vi "TCP Message Interpreter.vi"(8 "error in (no error)":errorcluster, 9 "Data":variant, 10 "Message":string, 11 "Guardian in":refnum<class "Guardian.lvclass">) -> (0 "error out":errorcluster, 3 "Guardian out":refnum<class "Guardian.lvclass">)   [LabVIEW 2026, in "TALOS.lvlib" / "Guardian.lvlib" / "Guardian.lvclass"]
doc: "Use this VI to send a message to the Guardian, from the outside (i.e. from a uService). For internal messages, use the Actor Framework messages system."
uses:
  Guardian.lvclass
  C:/LabVIEW Code/TALOS/builds/Actor Framework PPL/Actor Framework.lvlibp/1abvi3w/vi.lib/ActorFramework/Actor/Actor.lvclass
  C:/LabVIEW Code/TALOS/talos/Ancestor/Ancestor/Ancestor.lvclass
  Ancestor/Ancestor/Ancestor.lvclass/Ancestor.ctl
  Guardian Messages/Ready to launch Msg/Ready to launch Msg.lvclass/Ready to launch Msg.ctl
  Father of all uServices/Father of all uServices/Event Handler Items.ctl
  Guardian.lvclass/Guardian.ctl
  Guardian Messages/Message to uService Msg/Message to uService Msg.lvclass/Message to uService Msg.ctl
  Ancestor/Ancestor/Infinite Message Selector.ctl
  Guardian Messages/Message to Other Guardian Msg/Message to Other Guardian Msg.lvclass/Message to Other Guardian Msg.ctl
  Classes/uService List/uService List.lvclass/uService List.ctl
  Git Update Cluster.ctl
  builds/Actor Framework PPL/Actor Framework.lvlibp/1abvi3w/vi.lib/ActorFramework/Message Enqueuer/Message Priority.ctl
  Guardian Messages/Raise or Lower Abort Msg/Raise or Lower Abort Msg.lvclass/Raise or Lower Abort Msg.ctl
  Ancestor/Ancestor/Read Distr uS Map ref.vi
  Ancestor/Ancestor/Write Distr uS Map ref.vi
  Ancestor/Ancestor/Read ID.vi
  Read Guardian List.vi
  Write Guardian List.vi
  FGV/Error Memory/Get Error Description.vi
  Support VIs/Get PC name.vi
  Support VIs/Get Class Name.vi
  <vilib>/Utility/error.llb/Clear Errors.vi
  Support VIs/Circus Root Path.vi
  FGV/Error Memory/Error Memory Core.vi
  <vilib>/AdvancedString/Delimited String to 1D String Array.vi
  <vilib>/AdvancedString/Delimited String to 1D String Array (string).vi
  FGV/Error Memory/Error Crt Lvl checker.vi
  FGV/Error Memory/Error Memory Core.vi/40c8088d-b597-4017-91af-faa98e00292e.vi
  FGV/Error Memory/Error Memory Core.vi/d4a3ab98-063c-4e44-b43d-fbdcfe6c2be2.vi
  Support VIs/Global Memory.vi
  <vilib>/Utility/LVClass/Get LV Class Name.vi
  Support VIs/TALOS Root path.vi
  Support VIs/Read CSV worksheet.vi
  Support VIs/Global Constants.vi
  <vilib>/Utility/error.llb/General Error Handler.vi
  builds/Actor Framework PPL/Actor Framework.lvlibp/1abvi3w/vi.lib/ActorFramework/Message Enqueuer/Enqueue.vi
  Support VIs/Error Log.vi
  <vilib>/Utility/config.llb/Open Config Data.vi
  <vilib>/Utility/config.llb/Get Section Names.vi
  <vilib>/Utility/config.llb/Get Key Names.vi
  <vilib>/Utility/config.llb/Read Key.vi
  <vilib>/Utility/config.llb/Read Key (String).vi
  <vilib>/Utility/config.llb/Close Config Data.vi
  Ancestor/Ancestor/Ancestor.lvclass
  <vilib>/Comparison/Equal/Equal Functor/Equal Functor.lvclass
  Guardian Messages/Ready to launch Msg/Ready to launch Msg.lvclass
  Guardian Messages/Message to uService Msg/Message to uService Msg.lvclass
  Guardian Messages/Message to Other Guardian Msg/Message to Other Guardian Msg.lvclass
  Classes/Distributed uService Map/Distributed uService Map.lvclass
  Classes/Guardian List/Guardian List.lvclass
  Guardian Messages/Raise or Lower Abort Msg/Raise or Lower Abort Msg.lvclass
  builds/Actor Framework PPL/Actor Framework.lvlibp/1abvi3w/vi.lib/ActorFramework/Message Enqueuer/Message Enqueuer.lvclass
  TALOS.lvlib
  Father of all uServices/Father of all uServices/Father of all uServices.lvclass
  builds/Actor Framework PPL/Actor Framework.lvlibp/1abvi3w/vi.lib/ActorFramework/Actor/Actor.lvclass
  Im alive message.ctl
  Classes/uService List/uService List.lvclass
  Classes/Error Filter/Error Filter.lvclass
  FGV/Error Memory/Error Memory.lvlib
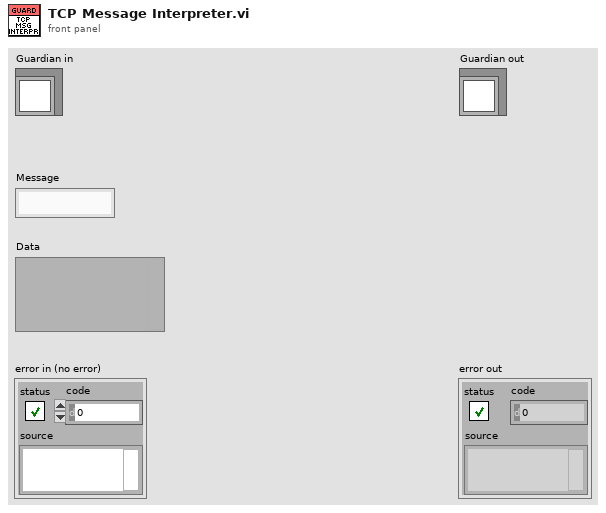
[diagram p1: front panel]
types:
  T1 = typedef "TALOS.lvlib/Father of all uServices.lvlib/Father of all uServices.lvclass/Event Handler Items.ctl" = enum16{"Button Pressed", "Message", "Ready to launch?", "Safe Mode", "Start RUN", "Stop RUN"}
  T2 = typedef "TALOS.lvlib/Ancestor.lvlib/Ancestor.lvclass/Infinite Message Selector.ctl" = enum16{"Start", "Stop", "Check", "Flush (Stop all)", "Init"}
  T3 = typedef "TALOS.lvlib/Guardian.lvlib/Guardian.lvclass/Im alive message.ctl" = cluster{"ID":string, "Time":timestamp, "Abort":bool, "Bearer":bool}
  T4 = typedef "Actor Framework.lvlibp/Message Enqueuer.lvclass/Message Priority.ctl" = enum16{"Low", "Normal", "High"}
  T5 = typedef "TALOS.lvlib/Guardian.lvlib/Guardian.lvclass/Git Update Cluster.ctl" = cluster{"branch name":string, "include critical PCs":bool, "update from git":bool}
  T6 = typedef "TALOS.lvlib/Guardian.lvlib/Guardian.lvclass/Run Config Data.ctl" = cluster{"Name":string, "uS List":string[]}
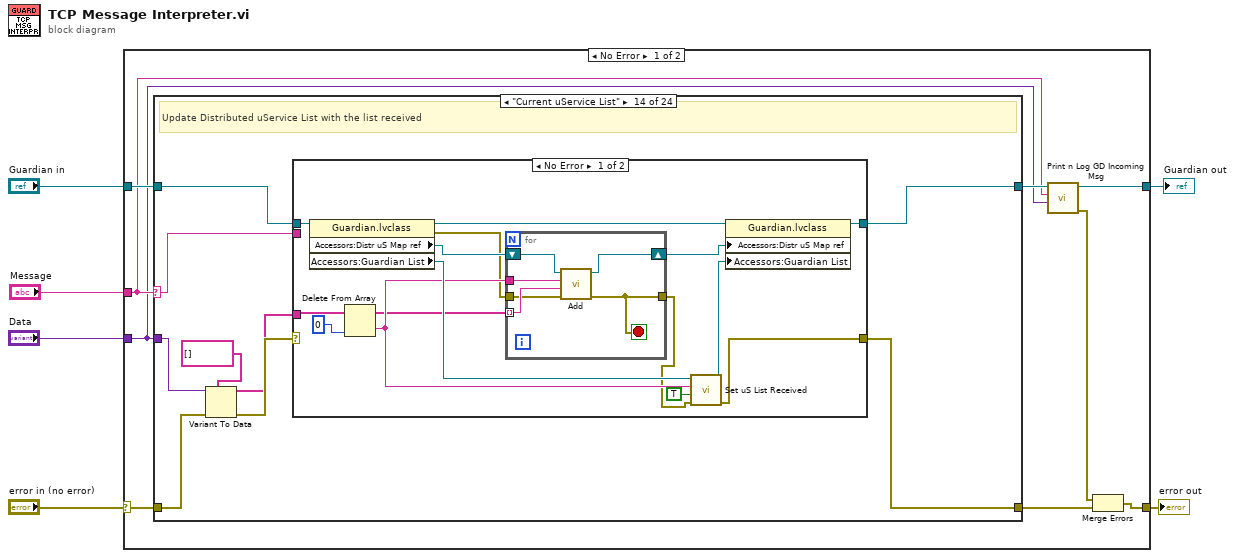
[diagram p0: block diagram]
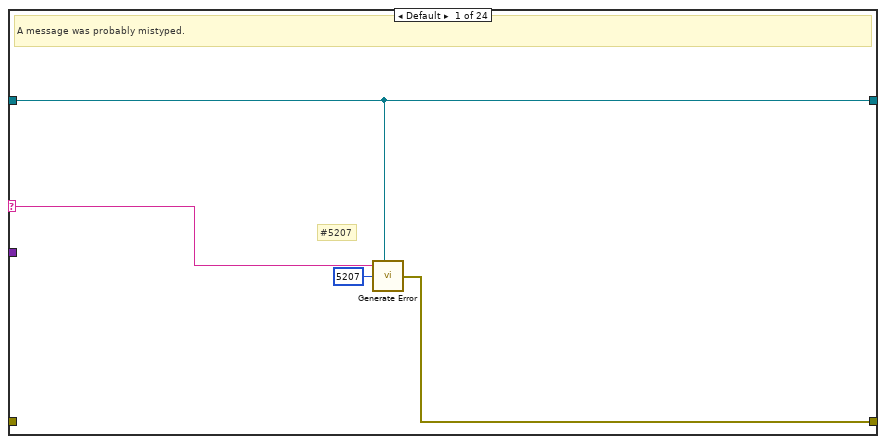
[diagram p2: hidden frame]
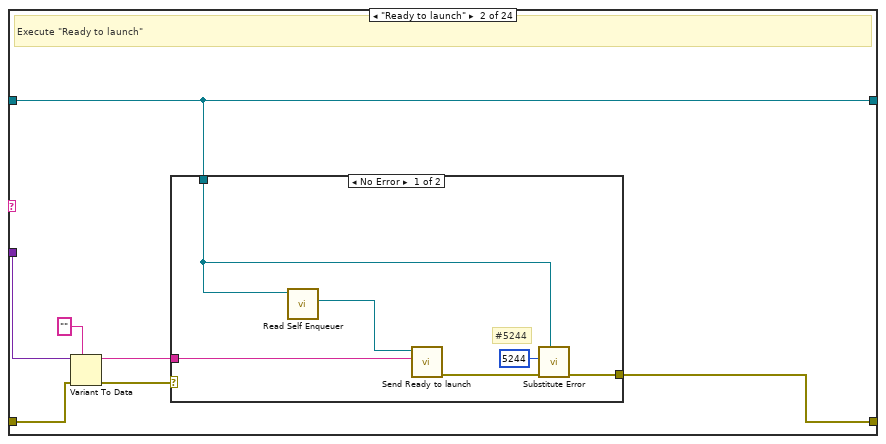
[diagram p3: hidden frame]
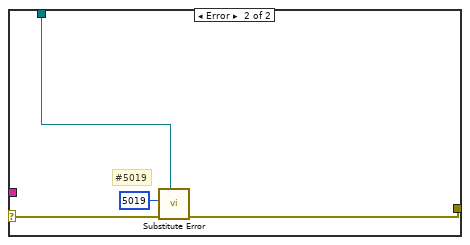
[diagram p4: hidden frame]
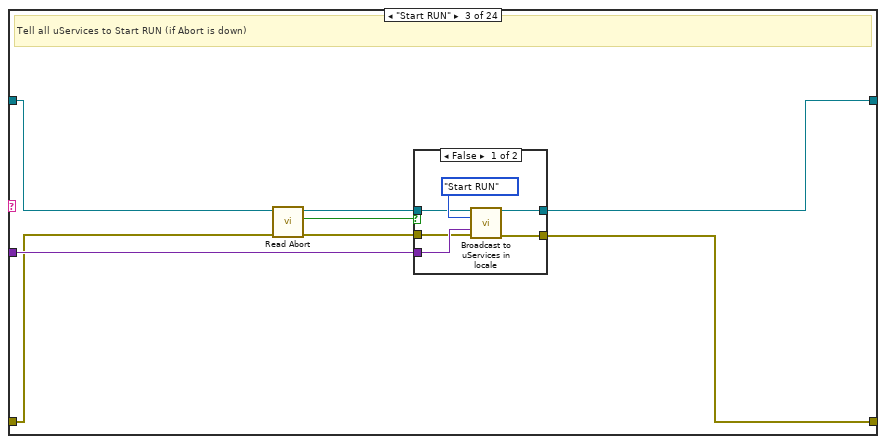
[diagram p5: hidden frame]
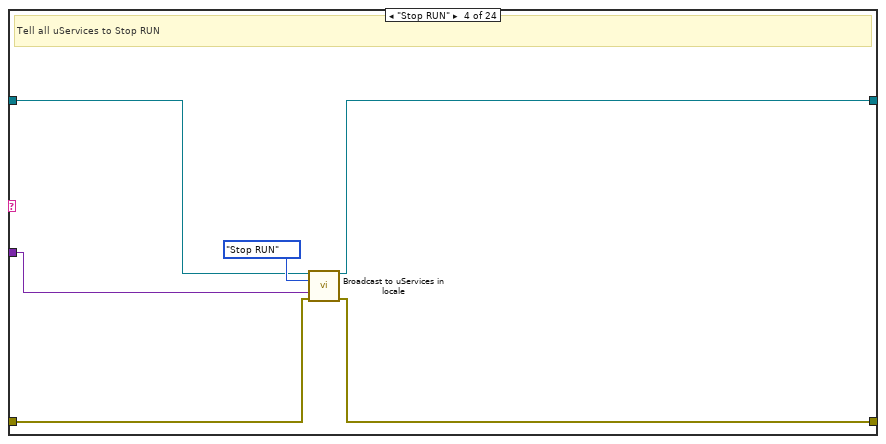
[diagram p7: hidden frame]
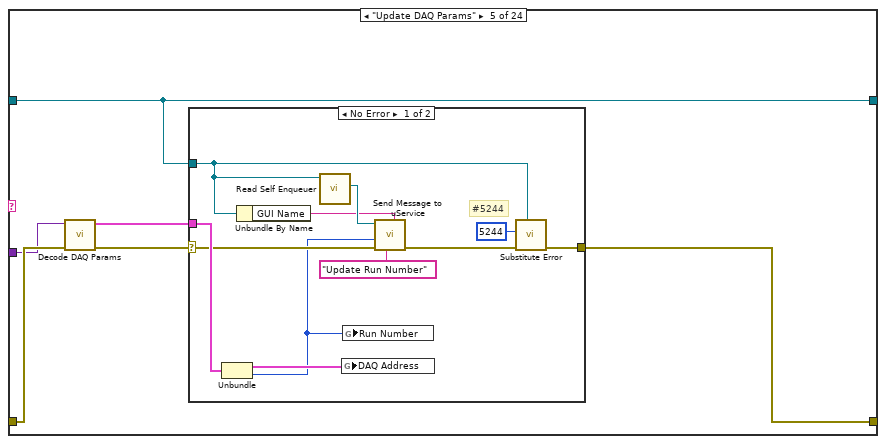
[diagram p8: hidden frame]
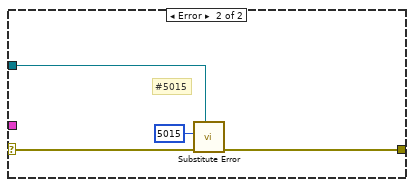
[diagram p9: hidden frame]
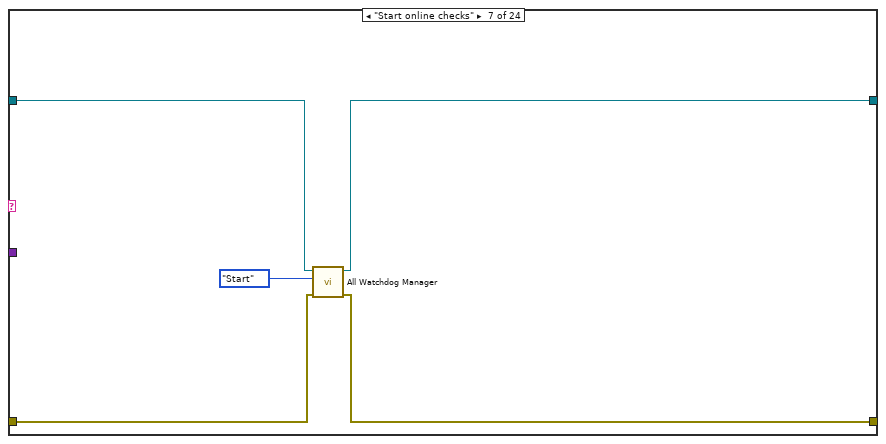
[diagram p11: hidden frame]
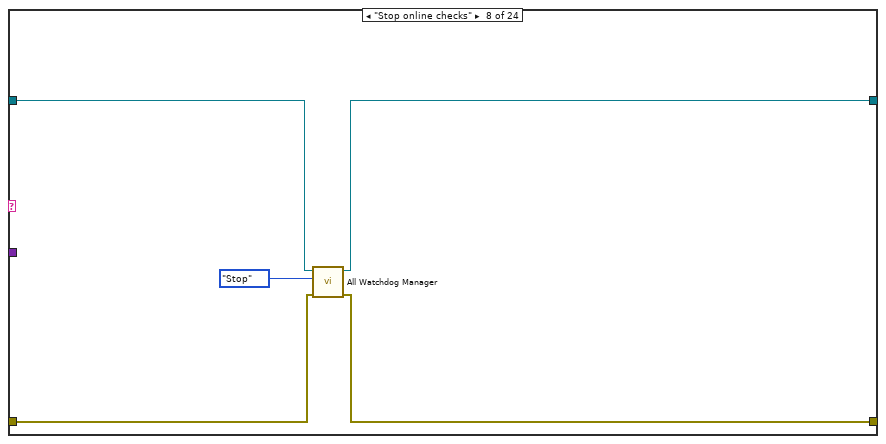
[diagram p12: hidden frame]
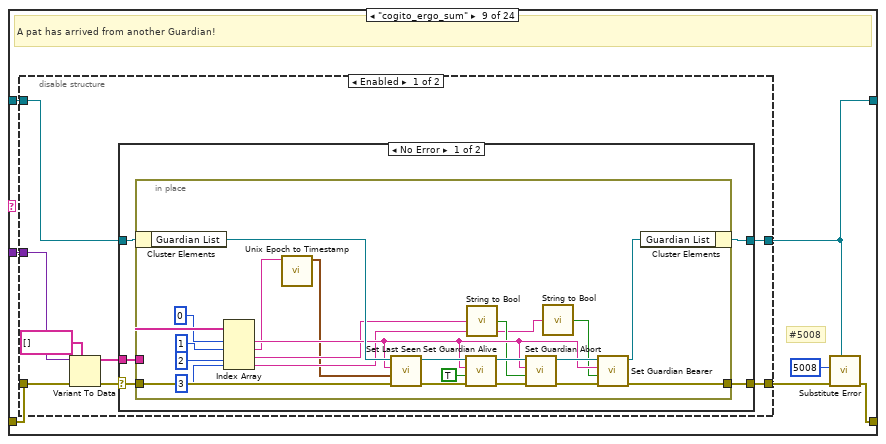
[diagram p13: hidden frame]
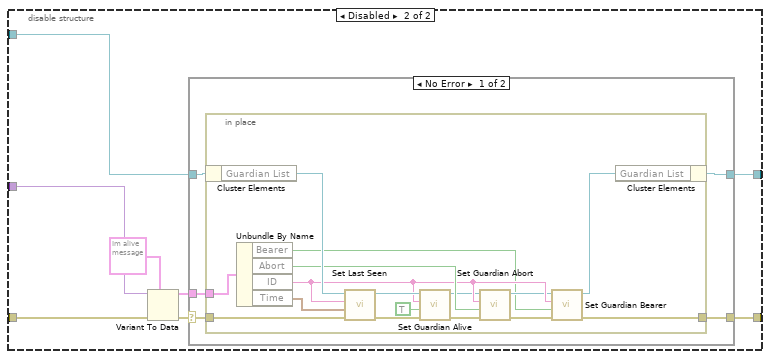
[diagram p15: hidden frame]
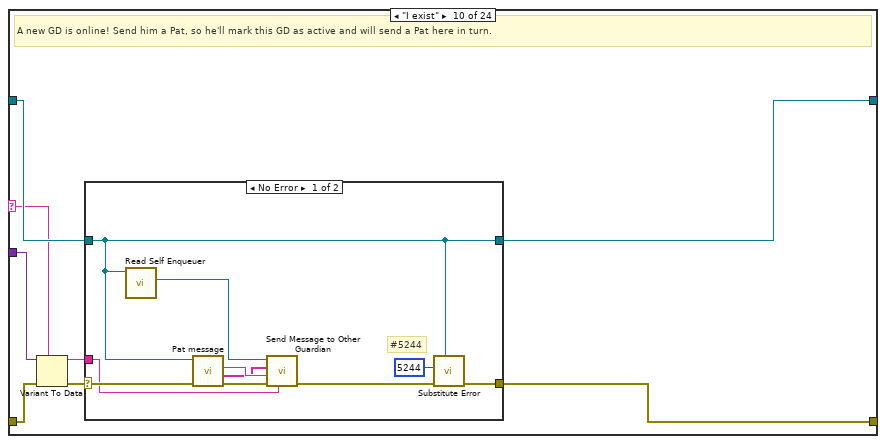
[diagram p17: hidden frame]
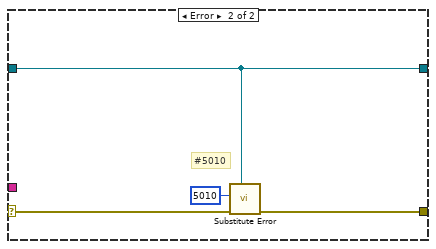
[diagram p18: hidden frame]
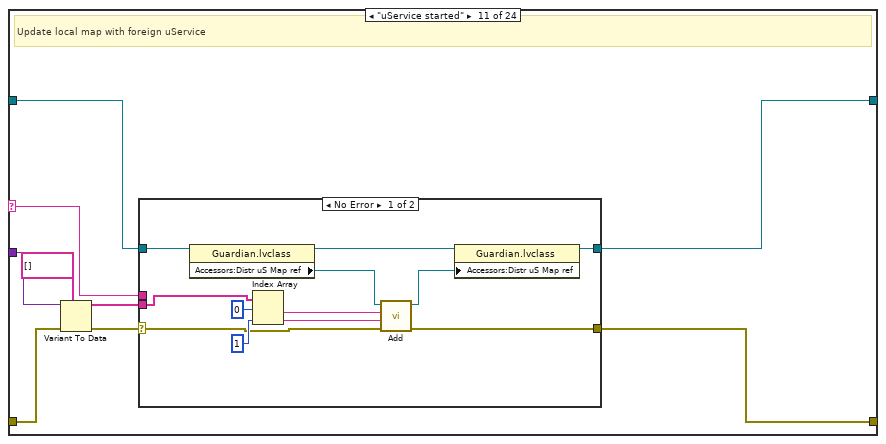
[diagram p19: hidden frame]
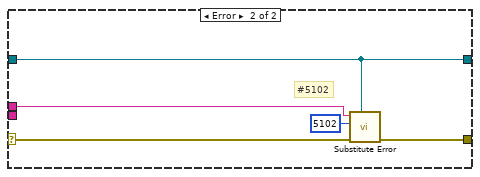
[diagram p20: hidden frame]
diagram:
  n1 = case shown="No Error" "error in (no error)" {
    selector: "error in (no error)" -> [w14 w499]
    tunnel: [w13 w499] -> w6
    tunnel: "Guardian in" -> [w12 w498]
    tunnel: [w10 w498] -> w3
    tunnel: "Data" -> [w8 _]
    tunnel: "Message" -> [w9 _]
    frame No Error {
      n2 = case shown="\"Current uService List\"" w9 {
        selector: w9 -> [w17 _ _ _ _ _ _ _ _ w169 w190 w216 w242 w272 _ w321 w330 w342 w351 _ _ _ w457 w495]
        tunnel: [w18 w25 w43 w56 w63 w80 w83 w88 w93 w168 w191 w217 w243 w274 w307 w315 w329 w341 w364 w375 w404 w410 w459 w493] -> w15
        tunnel: w8 -> [_ w24 w42 w53 w59 _ _ _ w98 w175 w196 w222 w248 w278 _ w319 w332 w344 w356 w368 w405 w417 w453 _]
        tunnel: w12 -> [w16 w26 w41 w54 w64 w81 w86 w91 w96 w171 w198 w224 w250 w280 w313 w314 w331 w343 w353 w374 w407 w412 w462 w496]
        tunnel: [w16 w26 w44 w57 w64 w81 w85 w90 w94 w170 w197 w223 w249 w279 w313 w314 w331 w343 w362 w372 w407 w411 w458 w494] -> w11
        tunnel: w14 -> [_ w23 w39 w55 w60 w80 w82 w87 w97 w174 w195 w221 w247 w277 w312 w318 w333 w345 w357 w369 w406 w416 w454 w497]
        frame Default {
          # "#5207"
          # "A message was probably mistyped."
          n3 = call "Generate Error.vi"("Optional String"=w17, "Class"=w16, "Error Code"=5207) -> ("error out"=w18:errorcluster)  [unwired: 4 in]
        }
        frame "Ready to launch" {
          # "Execute \"Ready to launch\""
          n4 = Variant To Data(error in=w23, type="", Variant=w24) -> (data=w20:string, error out=w21:errorcluster)
          n5 = case shown="No Error" w21 {
            selector: w21 -> [_ w35]
            tunnel: w26 -> [w27 w36]
            tunnel: [w28 w34] -> w25
            tunnel: w20 -> [w31 _]
            frame No Error {
              # "#5244"
              n6 = call "Read Self Enqueuer.vi"("Actor"=w27) -> ("Self Enqueuer"=w32:refnum<class "Message Enqueuer.lvclass">)  [unwired: 10 in]
              n7 = call "Send Ready to launch.vi"("GUID"=w31, "Message Enqueuer"=w32) -> ("error out"=w29:errorcluster)  [unwired: 8 in, 1 out]
              n8 = call "Substitute Error.vi"("LabVIEW Object"=w27, "error in (no error)"=w29, "Error Code"=5244) -> ("error out"=w28:errorcluster)  [unwired: 8 in]
            }
            frame Error {
              # "#5019"
              n9 = call "Substitute Error.vi"("LabVIEW Object"=w36, "error in (no error)"=w35, "Error Code"=5019) -> ("error out"=w34:errorcluster)  [unwired: 8 in]
            }
          }
        }
        frame "Start RUN" {
          # "Tell all uServices to Start RUN (if Abort is down)"
          n10 = call "Read Abort.vi"("error in (no error)"=w39, "Guardian in"=w41) -> ("error out"=w38:errorcluster, "Abort"=w37:bool, "Guardian out"=w40:refnum<class "Guardian.lvclass">)  [unwired: 7 in]
          n11 = case shown="False" w37 {
            tunnel: [w49 w52] -> w44
            tunnel: [w48 w51] -> w43
            tunnel: w42 -> [w47 _]
            tunnel: w40 -> [w46 w52]
            tunnel: w38 -> [w45 w51]
            frame False {
              n12 = call "Broadcast to uServices in locale.vi"("Guardian in"=w46, "Event type"=Event_Handler_Items."Start RUN", "Data"=w47, "error in (no error)"=w45) -> ("Guardian out"=w49:refnum<class "Guardian.lvclass">, "error out"=w48:errorcluster)  [unwired: 10 in]
            }
            frame True {
            }
          }
        }
        frame "Stop RUN" {
          # "Tell all uServices to Stop RUN"
          n13 = call "Broadcast to uServices in locale.vi"("Guardian in"=w54, "Event type"=Event_Handler_Items."Stop RUN", "Data"=w53, "error in (no error)"=w55) -> ("Guardian out"=w57:refnum<class "Guardian.lvclass">, "error out"=w56:errorcluster)  [unwired: 10 in]
        }
        frame "Update DAQ Params" {
          n14 = call "Decode DAQ Params.vi"("error in (no error)"=w60, "Data"=w59) -> ("error out"=w62:errorcluster, "Cluster"=w61:cluster{cluster{u16, string}, i32})  [unwired: 8 in]
          n15 = case shown="No Error" w62 {
            selector: w62 -> [w72 w79]
            tunnel: w61 -> [w73 _]
            tunnel: w64 -> [w66 w77]
            tunnel: [w65 w78] -> w63
            frame No Error {
              # "#5244"
              n16 = Unbundle(w73) -> (w70:cluster{u16, string}, w69:i32)
              n17 = Unbundle By Name(w66) -> ("GUI Name"=w74:string)
              n18 = call "Read Self Enqueuer.vi"("Actor"=w66) -> ("Self Enqueuer"=w75:refnum<class "Message Enqueuer.lvclass">)  [unwired: 10 in]
              n19 = global write "Global Memory.vi" "DAQ Address"(w70) -> ()
              n20 = global write "Global Memory.vi" "Run Number"(w69) -> ()
              n21 = call "Send Message to uService.vi"("uService ID"=w74, "Message"="Update Run Number", "error in (no error)"=w72, "Data"=w69, "Message Enqueuer"=w75) -> ("error out"=w67:errorcluster)  [unwired: 5 in, 1 out]
              n22 = call "Substitute Error.vi"("LabVIEW Object"=w66, "error in (no error)"=w67, "Error Code"=5244) -> ("error out"=w65:errorcluster)  [unwired: 8 in]
            }
            frame Error {
              # "#5015"
              n23 = call "Substitute Error.vi"("LabVIEW Object"=w77, "error in (no error)"=w79, "Error Code"=5015) -> ("error out"=w78:errorcluster)  [unwired: 8 in]
            }
          }
        }
        frame "Text Message" {
          # "For testing purpouses"
        }
        frame "Start online checks" {
          n24 = call "All Watchdog Manager.vi"("error in (no error)"=w82, "Infinite Message Selector"=Infinite_Message_Selector."Start", "Guardian in"=w86) -> ("error out"=w83:errorcluster, "Guardian out"=w85:refnum<class "Guardian.lvclass">)  [unwired: 6 in, 1 out]
        }
        frame "Stop online checks" {
          n25 = call "All Watchdog Manager.vi"("error in (no error)"=w87, "Infinite Message Selector"=Infinite_Message_Selector."Stop", "Guardian in"=w91) -> ("error out"=w88:errorcluster, "Guardian out"=w90:refnum<class "Guardian.lvclass">)  [unwired: 6 in, 1 out]
        }
        frame "cogito_ergo_sum" {
          # "#5008"
          # "A pat has arrived from another Guardian!"
          n26 = disable-structure shown="Enabled" {
            disable-tunnel: w98 -> [w106 w144]
            disable-tunnel: w97 -> [w105 w142]
            disable-tunnel: w96 -> [w102 w139]
            disable-tunnel: [w101 w138] -> w95
            disable-tunnel: [w100 w137] -> w94
            frame Enabled {
              n27 = Variant To Data(error in=w105, type=string[] [], Variant=w106) -> (data=w104:string[], error out=w103:errorcluster)
              n28 = case shown="No Error" w103 {
                selector: w103 -> [w108 w135]
                tunnel: w104 -> [w109 _]
                tunnel: w102 -> [w111 w136]
                tunnel: [w110 w136] -> w100
                tunnel: [w107 w135] -> w101
                frame No Error {
                  n29 = in-place {
                    in-place-border: w109 -> [w123]
                    in-place-border: w108 -> [w133]
                    in-place-border: [w125] -> w107
                    n30 = in-place-cluster #1(w111) -> ("Guardian List"=w134:refnum<class "Guardian List.lvclass">)
                    n31 = Index Array(array=w123, index #1=0 ("index"), index #2=1 ("index"), index #3=2 ("index"), index #4=3 ("index")) -> (element #1=w118:string, element #2=w112:string, element #3=w117:string, element #4=w115:string)
                    n32 = call "Unix Epoch to Timestamp.vi"("String"=w112) -> ("Time Stamp"=w113:timestamp)  [unwired: 10 in]
                    n33 = call-dynamic "Set Last Seen.vi"("error in (no error)"=w133, "Last Seen"=w113, "ID"=w118, "Guardian List in"=w134) -> ("error out"=w131:errorcluster, "Guardian List out"=w132:refnum<class "Guardian List.lvclass">)  [unwired: 6 in]
                    n34 = call-dynamic "Set Guardian Alive.vi"("error in (no error)"=w131, "Alive"=TRUE, "ID"=w118, "Guardian List in"=w132) -> ("error out"=w129:errorcluster, "Guardian List out"=w124:refnum<class "Guardian List.lvclass">)  [unwired: 6 in]
                    n35 = call "String to Bool.vi"("String"=w117) -> ("Boolean"=w116:bool)
                    n36 = call-dynamic "Set Guardian Abort.vi"("error in (no error)"=w129, "Abort"=w116, "ID"=w118, "Guardian List in"=w124) -> ("error out"=w128:errorcluster, "Guardian List out"=w127:refnum<class "Guardian List.lvclass">)  [unwired: 6 in]
                    n37 = call "String to Bool.vi"("String"=w115) -> ("Boolean"=w114:bool)
                    n38 = call-dynamic "Set Guardian Bearer.vi"("error in (no error)"=w128, "Bearer"=w114, "ID"=w118, "Guardian List in"=w127) -> ("error out"=w125:errorcluster, "Guardian List out"=w126:refnum<class "Guardian List.lvclass">)  [unwired: 6 in]
                    n39 = in-place-cluster #1("Guardian List"=w126) -> (w110:refnum<class "Guardian.lvclass">)
                  }
                }
                frame Error {
                }
              }
            }
            frame Disabled {
              n40 = Variant To Data(error in=w142, type=T3 {"ID"="", "Time"=timestamp(0 s since 1904-01-01), "Abort"=FALSE, "Bearer"=FALSE} ("cluster"), Variant=w144) -> (data=w141:T3, error out=w140:errorcluster)
              n41 = case shown="No Error" w140 {
                selector: w140 -> [w146 w166]
                tunnel: w141 -> [w147 _]
                tunnel: w139 -> [w149 w167]
                tunnel: [w148 w167] -> w137
                tunnel: [w145 w166] -> w138
                frame No Error {
                  n42 = in-place {
                    in-place-border: w147 -> [w164]
                    in-place-border: w146 -> [w162]
                    in-place-border: [w151] -> w145
                    n43 = in-place-cluster #2(w149) -> ("Guardian List"=w165:refnum<class "Guardian List.lvclass">)
                    n44 = Unbundle By Name(w164) -> ("Bearer"=w153:bool, "Abort"=w156:bool, "ID"=w155:string, "Time"=w163:timestamp)
                    n45 = call-dynamic "Set Last Seen.vi"("error in (no error)"=w162, "Last Seen"=w163, "ID"=w155, "Guardian List in"=w165) -> ("error out"=w160:errorcluster, "Guardian List out"=w161:refnum<class "Guardian List.lvclass">)  [unwired: 6 in]
                    n46 = call-dynamic "Set Guardian Alive.vi"("error in (no error)"=w160, "Alive"=TRUE, "ID"=w155, "Guardian List in"=w161) -> ("error out"=w158:errorcluster, "Guardian List out"=w150:refnum<class "Guardian List.lvclass">)  [unwired: 6 in]
                    n47 = call-dynamic "Set Guardian Abort.vi"("error in (no error)"=w158, "Abort"=w156, "ID"=w155, "Guardian List in"=w150) -> ("error out"=w157:errorcluster, "Guardian List out"=w154:refnum<class "Guardian List.lvclass">)  [unwired: 6 in]
                    n48 = call-dynamic "Set Guardian Bearer.vi"("error in (no error)"=w157, "Bearer"=w153, "ID"=w155, "Guardian List in"=w154) -> ("error out"=w151:errorcluster, "Guardian List out"=w152:refnum<class "Guardian List.lvclass">)  [unwired: 6 in]
                    n49 = in-place-cluster #2("Guardian List"=w152) -> (w148:refnum<class "Guardian.lvclass">)
                  }
                }
                frame Error {
                }
              }
            }
          }
          n50 = call "Substitute Error.vi"("LabVIEW Object"=w94, "error in (no error)"=w95, "Error Code"=5008) -> ("error out"=w93:errorcluster)  [unwired: 8 in]
        }
        frame "I exist" {
          # "A new GD is online! Send him a Pat, so he'll mark this GD as active and will send a Pat here in turn."
          n51 = Variant To Data(error in=w174, type=w169, Variant=w175) -> (data=w173:string, error out=w172:errorcluster)
          n52 = case shown="No Error" w172 {
            selector: w172 -> [w184 w188]
            tunnel: w173 -> [w183 _]
            tunnel: w171 -> [w177 w189]
            tunnel: [w177 w189] -> w170
            tunnel: [w176 w186] -> w168
            frame No Error {
              # "#5244"
              n53 = call "Read Self Enqueuer.vi"("Actor"=w177) -> ("Self Enqueuer"=w185:refnum<class "Message Enqueuer.lvclass">)  [unwired: 10 in]
              n54 = call "Pat message.vi"("error in (no error)"=w184, "Guardian in"=w177) -> ("error out"=w180:errorcluster, "Data"=w181:string[], "Message name"=w182:string)  [unwired: 6 in, 1 out]
              n55 = call "Send Message to Other Guardian.vi"("Guardian ID"=w183, "error in (no error)"=w180, "Message"=w182, "Data"=w181, "Message Enqueuer"=w185) -> ("error out"=w178:errorcluster)  [unwired: 5 in, 1 out]
              n56 = call "Substitute Error.vi"("LabVIEW Object"=w177, "error in (no error)"=w178, "Error Code"=5244) -> ("error out"=w176:errorcluster)  [unwired: 8 in]
            }
            frame Error {
              # "#5010"
              n57 = call "Substitute Error.vi"("LabVIEW Object"=w189, "error in (no error)"=w188, "Error Code"=5010) -> ("error out"=w186:errorcluster)  [unwired: 8 in]
            }
          }
        }
        frame "uService started" {
          # "Update local map with foreign uService"
          n58 = Variant To Data(error in=w195, type=string[] [], Variant=w196) -> (data=w192:string[], error out=w193:errorcluster)
          n59 = case shown="No Error" w193 {
            selector: w193 -> [w202 w215]
            tunnel: w198 -> [w199 w213]
            tunnel: [w210 w213] -> w197
            tunnel: w192 -> [w205 _]
            tunnel: [w209 w212] -> w191
            tunnel: w190 -> [_ w211]
            frame No Error {
              n60 = property class="Guardian.lvclass"(reference=w199) -> (reference out=w201:refnum<class "Guardian.lvclass">, "Accessors:Distr uS Map ref"=w200:refnum<data-value>)  [unwired: 1 in, 1 out]
              n61 = Index Array(array=w205, index #1=0 ("index"), index #2=1 ("index")) -> (element #1=w207:string, element #2=w206:string)
              n62 = call "Add.vi"("error in (no error)"=w202, "uService"=w206, "Guardian"=w207, "Distr uS Map ref in"=w200) -> ("error out"=w209:errorcluster, "Distr uS Map ref out"=w208:refnum<data-value>)  [unwired: 5 in, 1 out]
              n63 = property class="Guardian.lvclass"(reference=w201, "Accessors:Distr uS Map ref"=w208) -> (reference out=w210:refnum<class "Guardian.lvclass">)  [unwired: 1 in, 1 out]
            }
            frame Error {
              # "#5102"
              n64 = call "Substitute Error.vi"("LabVIEW Object"=w213, "error in (no error)"=w215, "Error Code"=5102, "Optional String"=w211) -> ("error out"=w212:errorcluster)  [unwired: 7 in]
            }
          }
        }
        frame "uService stopped" {
          # "Update local map with foreign uService"
          n65 = Variant To Data(error in=w221, type=string[] [], Variant=w222) -> (data=w218:string[], error out=w219:errorcluster)
          n66 = case shown="No Error" w219 {
            selector: w219 -> [w236 w241]
            tunnel: w224 -> [w226 w239]
            tunnel: [w225 w239] -> w223
            tunnel: w218 -> [w233 _]
            tunnel: [w230 w238] -> w217
            tunnel: w216 -> [_ w237]
            frame No Error {
              n67 = property class="Guardian.lvclass"(reference=w226) -> (reference out=w228:refnum<class "Guardian.lvclass">, "Accessors:Distr uS Map ref"=w227:refnum<data-value>)  [unwired: 1 in, 1 out]
              n68 = Index Array(array=w233, index #1=0 ("index"), index #2=1 ("index")) -> (element #1=w235:string, element #2=w234:string)
              n69 = call "Remove.vi"("error in (no error)"=w236, "uService ID"=w234, "Guardian"=w235, "Distr uS Map ref in"=w227) -> ("error out"=w230:errorcluster, "Distr uS Map ref out"=w229:refnum<data-value>)  [unwired: 5 in, 1 out]
              n70 = property class="Guardian.lvclass"(reference=w228, "Accessors:Distr uS Map ref"=w229) -> (reference out=w225:refnum<class "Guardian.lvclass">)  [unwired: 1 in, 1 out]
            }
            frame Error {
              # "#5102"
              n71 = call "Substitute Error.vi"("LabVIEW Object"=w239, "error in (no error)"=w241, "Error Code"=5102, "Optional String"=w237) -> ("error out"=w238:errorcluster)  [unwired: 7 in]
            }
          }
        }
        frame "Get uService List" {
          # "Give to the requesting Guardian the current uService List (for initialise the distributed one)"
          n72 = Variant To Data(error in=w247, type="", Variant=w248) -> (data=w244:string, error out=w245:errorcluster)
          n73 = case shown="No Error" w245 {
            selector: w245 -> [w261 w271]
            tunnel: w250 -> [w262 w269]
            tunnel: [w254 w269] -> w249
            tunnel: w244 -> [w266 _]
            tunnel: [w255 w268] -> w243
            tunnel: w242 -> [_ w267]
            frame No Error {
              # "requesting GD"
              # "#5244"
              n74 = call-dynamic "Access uService List.vi"("error in (no error)"=w261, "Ancestor in"=w262) -> ("error out"=w259:errorcluster, "uService List out"=w260:refnum<class "uService List.lvclass">, "Ancestor out"=w263:refnum<class "Guardian.lvclass">)  [unwired: 7 in]
              n75 = call "Get all IDs.vi"("error in (no error)"=w259, "uService List"=w260) -> ("error out"=w258:errorcluster, "All IDs"=w252:string[])  [unwired: 7 in, 1 out]
              n76 = property class="Guardian.lvclass"(reference=w263) -> (reference out=w254:refnum<class "Guardian.lvclass">, "Accessors:ID"=w251:string)  [unwired: 1 in, 1 out]
              n77 = Build Array (concatenate)(w251, w252) -> (w253:string[])
              n78 = call "Read Self Enqueuer.vi"("Actor"=w254) -> ("Self Enqueuer"=w265:refnum<class "Message Enqueuer.lvclass">)  [unwired: 10 in]
              n79 = call "Send Message to Other Guardian.vi"("Guardian ID"=w266, "error in (no error)"=w258, "Message"="Current uService List", "Data"=w253, "Message Enqueuer"=w265) -> ("error out"=w256:errorcluster)  [unwired: 5 in, 1 out]
              n80 = call "Substitute Error.vi"("LabVIEW Object"=w254, "error in (no error)"=w256, "Error Code"=5244) -> ("error out"=w255:errorcluster)  [unwired: 8 in]
            }
            frame Error {
              # "#5102"
              n81 = call "Substitute Error.vi"("LabVIEW Object"=w269, "error in (no error)"=w271, "Error Code"=5102, "Optional String"=w267) -> ("error out"=w268:errorcluster)  [unwired: 7 in]
            }
          }
        }
        frame "Current uService List" {
          # "Update Distributed uService List with the list received"
          n82 = Variant To Data(error in=w277, type=string[] [], Variant=w278) -> (data=w275:string[], error out=w276:errorcluster)
          n83 = case shown="No Error" w276 {
            selector: w276 -> [_ w306]
            tunnel: w280 -> [w293 w304]
            tunnel: [w292 w304] -> w279
            tunnel: w275 -> [w289 _]
            tunnel: [w281 w303] -> w274
            tunnel: w272 -> [_ w302]
            frame No Error {
              n84 = property class="Guardian.lvclass"(reference=w293) -> (reference out=w295:refnum<class "Guardian.lvclass">, error out=w284:errorcluster, "Accessors:Distr uS Map ref"=w287:refnum<data-value>, "Accessors:Guardian List"=w294:refnum<class "Guardian List.lvclass">)  [unwired: 1 in]
              n85 = Delete From Array(array=w289, index=0) -> (deleted portion=w286:string, array with subset deleted=w285:string[])  [unwired: 1 in]
              n86 = for {
                tunnel: w286 -> [w300]
                tunnel: w285 -> [w299] mode=indexing
                tunnel: w284 -> [w298]
                tunnel: [w297] -> w282
                shift-right: [w296] -> w283
                shift-left: w287 -> [w301]
                stop <- w297 stop-if-true
                n87 = call "Add.vi"("error in (no error)"=w298, "uService"=w299, "Guardian"=w300, "Distr uS Map ref in"=w301) -> ("error out"=w297:errorcluster, "Distr uS Map ref out"=w296:refnum<data-value>)  [unwired: 5 in, 1 out]
              }
              n88 = call-dynamic "Set uS List Received.vi"("error in (no error)"=w282, "uS List Received"=TRUE, "ID"=w286, "Guardian List in"=w294) -> ("error out"=w281:errorcluster, "Guardian List out"=w291:refnum<class "Guardian List.lvclass">)  [unwired: 6 in]
              n89 = property class="Guardian.lvclass"(reference=w295, "Accessors:Distr uS Map ref"=w283, "Accessors:Guardian List"=w291) -> (reference out=w292:refnum<class "Guardian.lvclass">)  [unwired: 1 in, 1 out]
            }
            frame Error {
              # "#5102"
              n90 = call "Substitute Error.vi"("LabVIEW Object"=w304, "error in (no error)"=w306, "Error Code"=5102, "Optional String"=w302) -> ("error out"=w303:errorcluster)  [unwired: 7 in]
            }
          }
        }
        frame "Reload INI files" {
          w310 = TRUE ("Load")
          # "Reload the configuration files"
          n91 = call "TALOS Config Param.vi"("Load"=w310, "error in (no error)"=w312) -> ("error out"=w311:errorcluster)  [unwired: 8 in, 1 out]
          n92 = call "Circus Config Param - Core.vi"("Load"=w310, "error in (no error)"=w311) -> ("error out"=w309:errorcluster)  [unwired: 8 in, 1 out]
          n93 = call "Errors Load.vi"("error in (no error)"=w309) -> ("error out"=w308:errorcluster)  [unwired: 10 in]
          n94 = call "Init.vi"("error in (no error)"=w308) -> ("error out"=w307:errorcluster)  [unwired: 10 in]
        }
        frame "Change Run LED color", "Reset Run LED", "Update Kasli Log" {
          # "It's OK, either is empty or is a string"
          # "#5244"
          n95 = Unbundle By Name(w314) -> ("GUI Name"=w322:string)
          n96 = call "Read Self Enqueuer.vi"("Actor"=w314) -> ("Self Enqueuer"=w323:refnum<class "Message Enqueuer.lvclass">)  [unwired: 10 in]
          n97 = call "Send Message to uService.vi"("uService ID"=w322, "Message"=w321, "error in (no error)"=w318, "Data"=w319, "Locale?"=TRUE, "Message Enqueuer"=w323) -> ("error out"=w316:errorcluster)  [unwired: 4 in, 1 out]
          n98 = call "Substitute Error.vi"("LabVIEW Object"=w314, "error in (no error)"=w316, "Error Code"=5244) -> ("error out"=w315:errorcluster)  [unwired: 8 in]
        }
        frame "Run Stopped with Errors" {
          # "#5244"
          # "Boolean encoded as a string"
          n99 = Unbundle By Name(w331) -> ("GUI Name"=w326:string)
          n100 = call "Read Self Enqueuer.vi"("Actor"=w331) -> ("Self Enqueuer"=w327:refnum<class "Message Enqueuer.lvclass">)  [unwired: 10 in]
          n101 = call "Send Message to uService.vi"("uService ID"=w326, "Message"=w330, "error in (no error)"=w333, "Data"=w332, "Locale?"=TRUE, "Message Enqueuer"=w327) -> ("error out"=w328:errorcluster)  [unwired: 4 in, 1 out]
          n102 = call "Substitute Error.vi"("LabVIEW Object"=w331, "error in (no error)"=w328, "Error Code"=5244) -> ("error out"=w329:errorcluster)  [unwired: 8 in]
        }
        frame "Update Error Listbox" {
          # "#5244"
          n103 = Unbundle By Name(w343) -> ("GUI Name"=w339:string)
          n104 = call "Decode Error Listbox.vi"("error in (no error)"=w345, "Data"=w344) -> ("error out"=w337:errorcluster, "Data out"=w336:variant)  [unwired: 8 in]
          n105 = call "Read Self Enqueuer.vi"("Actor"=w343) -> ("Self Enqueuer"=w338:refnum<class "Message Enqueuer.lvclass">)  [unwired: 10 in]
          n106 = call "Send Message to uService.vi"("uService ID"=w339, "Message"=w342, "error in (no error)"=w337, "Data"=w336, "Locale?"=TRUE, "Message Enqueuer"=w338) -> ("error out"=w340:errorcluster)  [unwired: 4 in, 1 out]
          n107 = call "Substitute Error.vi"("LabVIEW Object"=w343, "error in (no error)"=w340, "Error Code"=5244) -> ("error out"=w341:errorcluster)  [unwired: 8 in]
        }
        frame "Update Run Status" {
          # "#5260"
          # "#5244"
          n108 = Unbundle By Name(w353) -> ("GUI Name"=w352:string)
          n109 = call "Decode boolean.vi"("error in (no error)"=w357, "Data"=w356) -> ("error out"=w359:errorcluster, "Boolean"=w358:bool)  [unwired: 8 in]
          n110 = call "Read Self Enqueuer.vi"("Actor"=w353) -> ("Self Enqueuer"=w354:refnum<class "Message Enqueuer.lvclass">)  [unwired: 10 in]
          n111 = call "Send Message to uService.vi"("uService ID"=w352, "Message"=w351, "error in (no error)"=w359, "Data"=w358, "Locale?"=TRUE, "Message Enqueuer"=w354) -> ("error out"=w355:errorcluster)  [unwired: 4 in, 1 out]
          n112 = Variant To Data(type=TRUE ("Locale?"), Variant=w358) -> (data=w360:bool, error out=w361:errorcluster)  [unwired: 1 in]
          n113 = Bundle By Name(cluster=w353, "Run Status"=w360) -> (w362:refnum<class "Guardian.lvclass">)
          n114 = call "Substitute Error.vi"("LabVIEW Object"=w362, "error in (no error)"=w361, "Error Code"=5260) -> ("error out"=w348:errorcluster)  [unwired: 8 in]
          n115 = call "Substitute Error.vi"("LabVIEW Object"=w362, "error in (no error)"=w355, "Error Code"=5244) -> ("error out"=w363:errorcluster)  [unwired: 8 in]
          n116 = Merge Errors(w363, w348) -> (w364:errorcluster)
        }
        frame "Update from GIT" {
          (unwired) T5 {"branch name"="", "include critical PCs"=FALSE, "update from git"=FALSE} ("Git update cluster")
          n117 = call "Decode Update from Git.vi"("error in (no error)"=w369, "Data"=w368) -> ("error out"=w367:errorcluster, "branch name"=w366:string, "update from git"=w365:bool)  [unwired: 7 in]
          n118 = flat-sequence {
            tunnel: w367 -> [_]
            tunnel: [w376] -> w370
            tunnel: w374 -> [w383]
            tunnel: [w382] -> w371
            tunnel: w365 -> [w380]
            tunnel: w366 -> [w381]
            tunnel: w374 -> [w399]
            tunnel: [w398] -> w373
            tunnel: [w397] -> w372
            frame #0 {
              n119 = for {
                tunnel: i32[] [5004, 5005] ("Error Code") -> [w379] mode=indexing
                tunnel: [w378] -> w376 mode=indexing
                n120 = call "Add.vi"("Error Code"=w379) -> ("error out"=w378:errorcluster)  [unwired: 10 in]
              }
            }
            frame #1 {
              n121 = global read "Global Constants.vi" "Local"() -> (w387:bool)
              n122 = call "Is in Packed Library.vi"() -> ("error out"=w388:errorcluster, "Is In Packed Library"=w385:bool)  [unwired: 10 in]
              n123 = Not(x=w385) -> (.not. x?=w386:bool)
              n124 = Or(x=w387, y=w386) -> (x .or. y?=w384:bool)
              n125 = case shown="False" w384 {
                tunnel: w388 -> [w393 w396]
                tunnel: [w392 w395] -> w382
                tunnel: w383 -> [w391 _]
                tunnel: w380 -> [w390 _]
                tunnel: w381 -> [w389 _]
                frame False {
                  n126 = call "Launch Update from Git.vi"("error in (no error)"=w393, "Branch name"=w389, "Update GIT"=w390, "Guardian in"=w391) -> ("error out"=w392:errorcluster)  [unwired: 6 in, 1 out]
                }
                frame True {
                  n127 = call "Temporised Pop-up Window.vi"("error in (no error)"=w396, "Text"="I'm dying!") -> ("error out"=w395:errorcluster)  [unwired: 9 in]
                }
              }
            }
            frame #2 {
              n128 = call "System shutdown.vi"("Guardian in"=w399) -> ("error out"=w398:errorcluster, "Guardian out"=w397:refnum<class "Guardian.lvclass">)  [unwired: 9 in]
            }
          }
          n129 = Merge Errors(w373, w371, w370) -> (w375:errorcluster)
        }
        frame "4b0rt" {
          # "I don't throw an error here because it will likely cause a loop"
          # "#5244"
          # "Directly run the \"Raise/Lower Abort\" VI creates a recursive loop, so need ot call it as a message."
          n130 = call "Decode ABORT Message.vi"("error in (no error)"=w406, "Data"=w405) -> ("Sender"=w401:string, "Abort"=w400:bool)  [unwired: 8 in]
          n131 = call "Read Self Enqueuer.vi"("Actor"=w407) -> ("Self Enqueuer"=w409:refnum<class "Message Enqueuer.lvclass">)  [unwired: 10 in]
          n132 = call "Send Raise or Lower Abort.vi"("Message Priority (Normal)"=Message_Priority."High", "Sender"=w401, "New Abort Value"=w400, "Message Enqueuer"=w409) -> ("error out"=w403:errorcluster)  [unwired: 6 in, 1 out]
          n133 = call "Substitute Error.vi"("LabVIEW Object"=w407, "error in (no error)"=w403, "Error Code"=5244) -> ("error out"=w404:errorcluster)  [unwired: 8 in]
        }
        frame "Ladies and Gentlemen it has been a pleasure" {
          # "Strip the Guardian from the list of the active ones, to avoid entering into Abort."
          n134 = Variant To Data(error in=w416, type="", Variant=w417) -> (data=w413:string, error out=w414:errorcluster)
          n135 = case shown="No Error" w414 {
            selector: w414 -> [w426 w452]
            tunnel: w413 -> [w427 w449]
            tunnel: w412 -> [w428 w450]
            tunnel: [w423 w450] -> w411
            tunnel: [w424 w448] -> w410
            frame No Error {
              w425 = 5053  # #5053
              n136 = in-place {
                in-place-border: w427 -> [w437]
                in-place-border: w426 -> [w436]
                in-place-border: [w434] -> w419
                in-place-border: [w437] -> w418
                n137 = in-place-cluster #3(w428) -> ("Guardian List"=w439:refnum<class "Guardian List.lvclass">)
                n138 = call-dynamic "Set Guardian Alive.vi"("error in (no error)"=w436, "Alive"=FALSE, "ID"=w437, "Guardian List in"=w439) -> ("error out"=w431:errorcluster, "Guardian List out"=w430:refnum<class "Guardian List.lvclass">)  [unwired: 6 in]
                n139 = call-dynamic "Set uS List Received.vi"("error in (no error)"=w431, "uS List Received"=FALSE, "ID"=w437, "Guardian List in"=w430) -> ("error out"=w433:errorcluster, "Guardian List out"=w432:refnum<class "Guardian List.lvclass">)  [unwired: 6 in]
                n140 = disable-structure shown="Disabled" {
                  disable-tunnel: w432 -> [w445 w447]
                  disable-tunnel: [w444 w447] -> w438
                  disable-tunnel: w437 -> [w443 _]
                  disable-tunnel: w433 -> [w442 w446]
                  disable-tunnel: [w440 w446] -> w434
                  frame Disabled {
                    n141 = call-dynamic "Set Last Seen.vi"("error in (no error)"=w442, "Last Seen"=timestamp(-3600 s since 1904-01-01) ("y"), "ID"=w443, "Guardian List in"=w445) -> ("error out"=w440:errorcluster, "Guardian List out"=w444:refnum<class "Guardian List.lvclass">)  [unwired: 6 in]
                  }
                  frame Enabled {
                  }
                }
                n142 = in-place-cluster #3("Guardian List"=w438) -> (w421:refnum<class "Guardian.lvclass">)
              }
              n143 = property class="Guardian.lvclass"(reference=w421) -> (reference out=w423:refnum<class "Guardian.lvclass">, "Accessors:Distr uS Map ref"=w422:refnum<data-value>)  [unwired: 1 in, 1 out]
              n144 = call "Remove Guardian.vi"("error in (no error)"=w419, "Guardian ID"=w418, "Distr uS Map ref in"=w422) -> ("error out"=w420:errorcluster)  [unwired: 7 in, 1 out]
              n145 = call "Substitute Error.vi"("LabVIEW Object"=w423, "error in (no error)"=w420, "Error Code"=w425) -> ("error out"=w424:errorcluster)  [unwired: 8 in]
            }
            frame Error {
              w451 = 5207  # #5207
              n146 = call "Substitute Error.vi"("LabVIEW Object"=w450, "error in (no error)"=w452, "Error Code"=w451, "Optional String"=w449) -> ("error out"=w448:errorcluster)  [unwired: 7 in]
            }
          }
        }
        frame "Add uSs from Config", "Change Run Config", "Realign uSs from Config" {
          w461 = 5056  # #5056
          # "Load the new Run Config file, stop and launch uServices accordingly."
          n147 = call "Run Config Data Decoder.vi"("error in (no error)"=w454, "Data"=w453) -> ("error out"=w456:errorcluster, "Run Config Data"=w455:T6)  [unwired: 8 in]
          n148 = case shown="No Error" w456 {
            selector: w456 -> [w471 w490]
            tunnel: w455 -> [w472 _]
            tunnel: w462 -> [w473 w489]
            tunnel: [w463 w490] -> w460
            tunnel: [w464 w489] -> w458
            tunnel: w457 -> [w468 _]
            frame No Error {
              n149 = Unbundle By Name(w472) -> ("Name"=w470:string, "uS List"=w466:string[])
              n150 = Unbundle By Name(w473) -> ("GUI Name"=w475:string)
              n151 = call "Read Self Enqueuer.vi"("Actor"=w473) -> ("Self Enqueuer"=w476:refnum<class "Message Enqueuer.lvclass">)  [unwired: 10 in]
              n152 = Bundle By Name(cluster=w473, "Run Config Data"=w472) -> (w465:refnum<class "Guardian.lvclass">)
              n153 = call "Send Message to uService.vi"("uService ID"=w475, "Message"="Update Run Config", "error in (no error)"=w471, "Data"=w470, "Locale?"=TRUE, "Message Enqueuer"=w476) -> ("error out"=w467:errorcluster)  [unwired: 4 in, 1 out]
              n154 = case shown="\"Realign uSs from Config\"" w468 {
                tunnel: w467 -> [w477 w483 w488]
                tunnel: w466 -> [_ w482 w486]
                tunnel: w465 -> [w478 w481 w485]
                tunnel: [w478 w480 w484] -> w464
                tunnel: [w477 w479 w487] -> w463
                frame "Change Run Config", Default {
                  # "Do nothing on uSs."
                }
                frame "Add uSs from Config" {
                  n155 = call "Add uSs from Run Config.vi"("error in (no error)"=w483, "uS List"=w482, "Guardian in"=w481) -> ("error out"=w479:errorcluster, "Guardian out"=w480:refnum<class "Guardian.lvclass">)  [unwired: 7 in]
                }
                frame "Realign uSs from Config" {
                  n156 = call "Realign uSs from Run Config.vi"("error in (no error)"=w488, "uS List"=w486, "Guardian in"=w485) -> ("error out"=w487:errorcluster, "Guardian out"=w484:refnum<class "Guardian.lvclass">)  [unwired: 7 in]
                }
              }
            }
            frame Error {
            }
          }
          n157 = call "Substitute Error.vi"("LabVIEW Object"=w458, "error in (no error)"=w460, "Error Code"=w461) -> ("error out"=w459:errorcluster)  [unwired: 8 in]
        }
        frame "Dismiss All Errors" {
          n158 = call "Get Local Error Manager Name.vi"() -> ("Error Manager ID"=w491:string)  [unwired: 1 in]
          n159 = call "Message to uService.vi"("Guardian in"=w496, "uService ID"=w491, "Message"=w495, "error in (no error)"=w497, "Locale?"=TRUE) -> ("Guardian out"=w494:refnum<class "Guardian.lvclass">, "error out"=w493:errorcluster)  [unwired: 9 in]
        }
      }
      n160 = call "Print n Log GD Incoming Msg.vi"("Data"=w8, "Message"=w9, "Guardian in"=w11) -> ("error out"=w7:errorcluster, "Guardian out"=w10:refnum<class "Guardian.lvclass">)  [unwired: 7 in]
      n161 = Merge Errors(w7, w15) -> (w13:errorcluster)
    }
    frame Error {
    }
  }
  "error out" <- w6
  "Guardian out" <- w3
